vi "Set Transactions.vi"(8 "error in (no error)":errorcluster, 10 "Transactions":refnum<class "Transaction.lvclass">[](array[class]), 11 "Statement in":refnum<class "Statement.lvclass">) -> (0 "error out":errorcluster, 3 "Statement out":refnum<class "Statement.lvclass">)   [LabVIEW 2018, in "Statement.lvclass"]
uses:
  Statement.lvclass
  Transaction/Transaction.lvclass
  Statement.lvclass/Statement.ctl
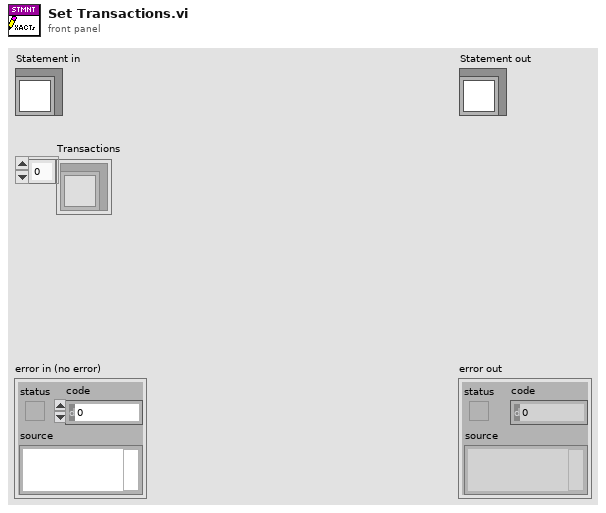
[diagram p1: front panel]
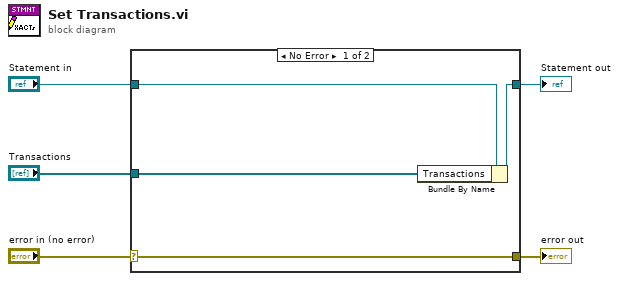
[diagram p0: block diagram]
diagram:
  n1 = case shown="No Error" "error in (no error)" {
    selector: "error in (no error)" -> [w9 w10]
    tunnel: [w9 w10] -> w4
    tunnel: [w7 w11] -> w2
    tunnel: "Statement in" -> [w8 w11]
    tunnel: "Transactions" -> [w6 _]
    frame No Error {
      n2 = Bundle By Name(cluster=w8, "Transactions"=w6) -> (w7:refnum<class "Statement.lvclass">)
    }
    frame Error {
    }
  }
  "error out" <- w4
  "Statement out" <- w2
